vi "Player Info.vi"(11 "Atom in":refnum<class "Atom.lvclass">) -> (0 "Defeat Speech":string="ggwp", 1 "Victory Speech":string="I am become death, the destroyer of worlds.", 2 "Name":string="Atom", 3 "Atom out":refnum<class "Atom.lvclass">)   [LabVIEW 2020, in "Atom.lvclass"]
uses:
  Atom.lvclass
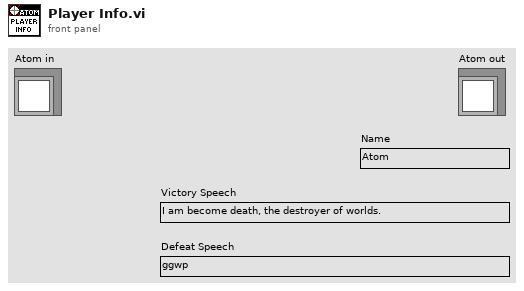
[diagram p1: front panel]
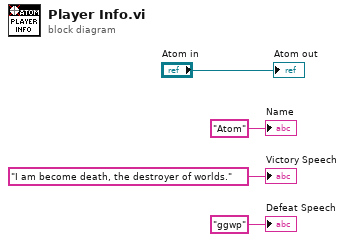
[diagram p0: block diagram]
diagram:
  "Atom out" <- "Atom in"
  "Name" <- "Atom" ("Name")
  "Victory Speech" <- "I am become death, the destroyer of worlds." ("Victory Speech")
  "Defeat Speech" <- "ggwp" ("Defeat Speech")
